vi "test.vi"() -> ()   [LabVIEW 2010]
uses:
  XUserDropdown.xctl
panel:
  in  "stop":bool
  out "currently selected user":string
  in  "user":string(xcontrol)
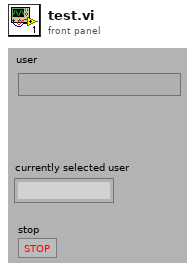
[diagram p1: front panel]
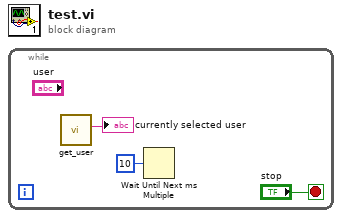
[diagram p0: block diagram]
diagram:
  n1 = while {
    stop <- "stop" stop-if-true
    n2 = call "get_user.vi"() -> ("username out"=→"currently selected user":string)  [unwired: 10 in, 1 out]
    n3 = Wait Until Next ms Multiple(millisecond multiple=u32 10) -> ()  [unwired: 1 out]
  }
